vi "lab3.vi"() -> ()   [LabVIEW 2019]
uses:
  <vilib>/imath/engines/lvmath2/RunTimeEngine/BuiltInFunctions/iir_elliptic/NIMS_[2o]_iir_elliptic(I32,DBL2,V,Str).vi
  <vilib>/imath/engines/lvmath2/RunTimeEngine/ErrorHandling/NIMS_Create Error From Enums.vi
  <vilib>/imath/engines/lvmath/Plug In/Control Design/BuiltInFunctions/tf/NIMS_CD_tf(num,den,Ts).vi
  <vilib>/imath/engines/lvmath2/RunTimeEngine/BuiltInFunctions/iir_elliptic/NIMS_[3o]_iir_elliptic(I32,DBL2,V,Str).vi
  <vilib>/imath/engines/lvmath/Plug In/Control Design/BuiltInFunctions/zpk/NIMS_CD_zpk(zeros,poles,k,Ts).vi
  <vilib>/imathl/engines/lvmath/Functions/Error Handling/Create Error.vi
  <vilib>/imath/engines/lvmath2/RunTimeEngine/BuiltInFunctions/iir_elliptic/NIMS_[4o]_iir_elliptic(I32,DBL2,V,Str).vi
  <vilib>/imath/engines/lvmath/Plug In/Control Design/BuiltInFunctions/ss/NIMS_CD_ss(A,B,C,D).vi
  <vilib>/imath/engines/lvmath2/RunTimeEngine/NodeEndStatement/NIMS_NodeEndStatement_Output.vi
  <instcachedir>/0/NIMS_NodeEndStatement_Output_53EC0D466D134D7ABD903AC30B43404B.lvgen/NIMS_NodeEndStatement_Output_53EC0D466D134D7ABD903AC30B43404B_011.vi
  <instcachedir>/0/NIMS_NodeEndStatement_Output_53EC0D466D134D7ABD903AC30B43404B.lvgen/NIMS_NodeEndStatement_Output_53EC0D466D134D7ABD903AC30B43404B_010.vi
  <instcachedir>/0/NIMS_NodeEndStatement_Output_53EC0D466D134D7ABD903AC30B43404B.lvgen/NIMS_NodeEndStatement_Output_53EC0D466D134D7ABD903AC30B43404B_009.vi
  <vilib>/imath/engines/lvmath2/RunTimeEngine/ErrorHandling/NIMS_Finalize Error.vi
  <vilib>/addons/Control Design/_Time Response Analysis/Time Response.llb/Time Response subVI/cd_Step Response (State-Space).vi
  <vilib>/addons/Control Design/_Frequency Response Analysis/Frequency Response.llb/Frequency Response subVI/cd_Bode (State Space).vi
  <vilib>/addons/Control Design/_Utility/Model Viewer.llb/Model Viewer SubVI/cd_Draw State-Space Equation (SS).vi
  <vilib>/addons/Control Design/_Frequency Response Analysis/Frequency Response.llb/Frequency Response subVI/cd_Bode (Zero-Pole-Gain).vi
  <vilib>/addons/Control Design/_Time Response Analysis/Time Response.llb/Time Response subVI/cd_Step Response (Zero-Pole-Gain).vi
  <vilib>/addons/Control Design/_Utility/Model Viewer.llb/Model Viewer SubVI/cd_Draw Zero-Pole-Gain Equation (ZPK).vi
  <vilib>/addons/Control Design/_Frequency Response Analysis/Frequency Response.llb/Frequency Response subVI/cd_Bode (Transfer Function).vi
  <vilib>/addons/Control Design/_Time Response Analysis/Time Response.llb/Time Response subVI/cd_Step Response (Transfer Function).vi
  <vilib>/addons/Control Design/_Utility/Model Viewer.llb/Model Viewer SubVI/cd_Draw Transfer Function Equation (TF).vi
  <vilib>/addons/Control Design/_Utility/NI_CD_Model Viewer.lvlib
  <vilib>/addons/Control Design/_Time Response Analysis/NI_CD_Time Response.lvlib
  <vilib>/addons/Control Design/_Frequency Response Analysis/NI_CD_Frequency Response.lvlib
panel:
  out "Нули, полюса и коэффициент усиления (zpk)":picture
  out "Реакция на ступенчатое воздействие":cluster{"time":dbl[], dbl[]}[](graph)
  out "Реакция АЧХ, реализованных различным способом":cluster{"time":dbl[], dbl[]}[](graph)
  out "АЧХ":cluster{"time":dbl[], dbl[]}[](graph)
  out "Погрешность реакции на ступенчатое воздействие":cluster{"time":dbl[], dbl[]}[](graph)
  out "Передаточная функция":picture
  out "Модель в пространстве состояний":picture
  in  "dbp":dbl
  in  "n":dbl
  in  "dbs":dbl
  in  "w":dbl
  in  "Time Range":cluster{"t0":dbl, "dt":dbl, "tf":dbl}
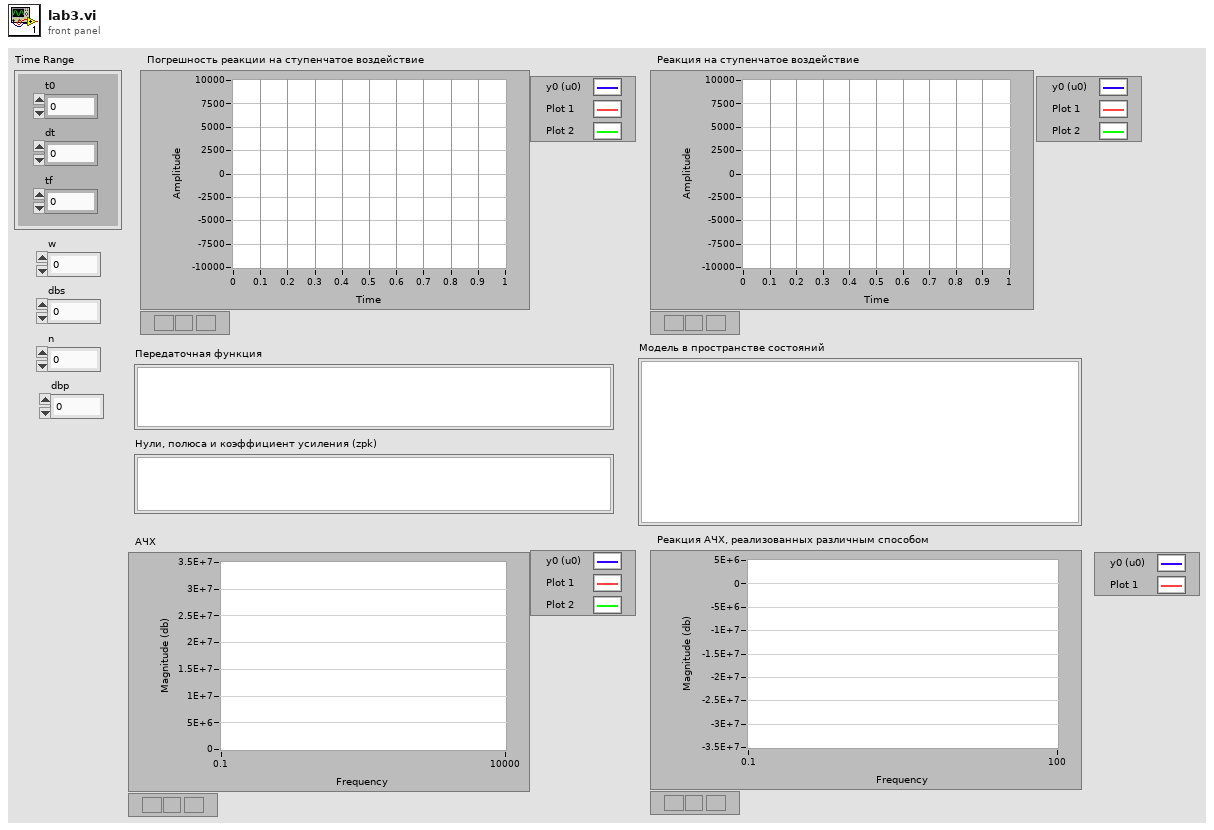
[diagram p1: front panel]
types:
  T1 = typedef "NI_LinSys_Model Typedefs.lvlib/CD Transfer Function Model (MIMO).ctl" = cluster{"properties":T2, "transfer function(s)":T3[][]}
  T2 = typedef "NI_LinSys_Model Typedefs.lvlib/CD General Elements.ctl" = cluster{"Model name":string, "Input names":string[], "Output names":string[], "Input Delays":dbl[], "Output Delays":dbl[], "Sampling Time":dbl, "Notes":string}
  T3 = typedef "NI_LinSys_Model Typedefs.lvlib/CD Transfer Function Model (SISO).ctl" = cluster{"Numerator":dbl[], "Denominator":dbl[], "delay":dbl}
  T4 = typedef "NI_LinSys_Model Typedefs.lvlib/CD Zero-Pole-Gain Model (MIMO).ctl" = cluster{"properties":T2, "zero-pole-gain(s)":T5[][]}
  T5 = typedef "NI_LinSys_Model Typedefs.lvlib/CD Zero-Pole-Gain Model (SISO).ctl" = cluster{"Gain":dbl, "Zeros":cdb[], "Poles":cdb[], "delay":dbl}
  T6 = typedef "NI_LinSys_Model Typedefs.lvlib/CD State Space Model (MIMO).ctl" = cluster{"properties":T2, "A":dbl[][], "B":dbl[][], "C":dbl[][], "D":dbl[][], "StateNames":string[], "Transport Delay":dbl[][]}
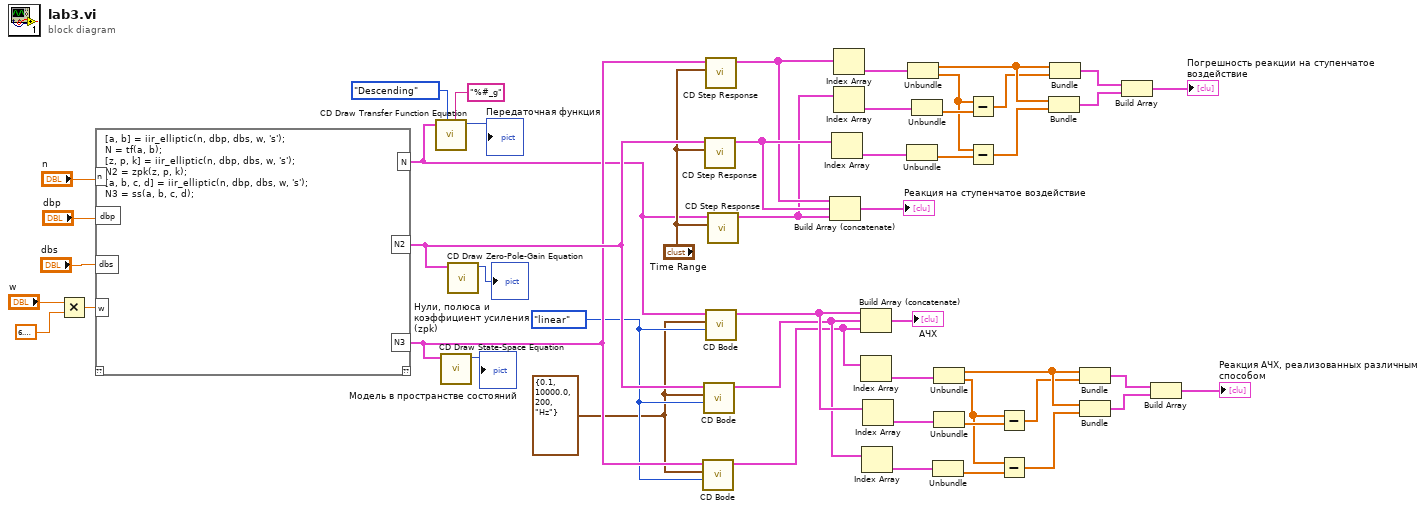
[diagram p0: block diagram]
diagram:
  w35 = enum16{"linear"}."linear"
  w34 = cluster{dbl, dbl, i32, enum16{"Hz"}} {0.1, 10000.0, 200, enum."Hz"} ("Frequency Range")
  n1 = Multiply(x="w", y=6.283185307179586) -> (x*y=w48:dbl)
  n2 = mathscript code="[a, b] = iir_elliptic(n, dbp, dbs, w, 's');\nN = tf(a, b);\n[z, p, k] = iir_elliptic(n, dbp, dbs, w, 's');\nN2 = zpk(z, p, k);\n[a, b, c, d] = iir_elliptic(n, dbp, dbs, w, 's');\nN3 = ss(a, b, c, d);"("n"="n", "dbp"="dbp", "dbs"="dbs", "w"=w48) -> ("N"=w36:T1, "N2"=w43:T4, "N3"=w37:T6)  [unwired: 1 in, 1 out]
  n3 = call-poly <vilib>:"CD Draw Transfer Function Equation.vi"("Format Coefficients"="%#_g", "Display Format"=enum16{"", "Ascending", "Descending"}."Descending", "Transfer Function Model"=w36) -> ("Equation"=→"Передаточная функция":picture)  [unwired: 6 in, 2 out]
  n4 = call-poly <vilib>:"CD Draw State-Space Equation.vi"("State-Space Model"=w37) -> ("Equation"=→"Модель в пространстве состояний":picture)  [unwired: 8 in, 2 out]
  n5 = call-poly <vilib>:"CD Draw Zero-Pole-Gain Equation.vi"("Zero-Pole-Gain Model"=w43) -> ("Equation"=→"Нули, полюса и коэффициент усиления (zpk)":picture)  [unwired: 8 in, 2 out]
  n6 = call-poly <vilib>:"CD Bode.vi"("Magnitude Scale"=w35, "Frequency Range"=w34, "State-Space Model"=w37) -> ("Bode Magnitude"=w22:cluster{"W":dbl[], "Magnitude":dbl[]}[])  [unwired: 4 in, 4 out]
  n7 = call-poly <vilib>:"CD Bode.vi"("Magnitude Scale"=w35, "Frequency Range"=w34, "Zero-Pole-Gain Model"=w43) -> ("Bode Magnitude"=w23:cluster{"W":dbl[], "Magnitude":dbl[]}[])  [unwired: 4 in, 4 out]
  n8 = call-poly <vilib>:"CD Step Response.vi"("Time Range"="Time Range", "Zero-Pole-Gain Model"=w43) -> ("Step Response Graph"=w3:cluster{"time":dbl[], dbl[]}[])  [unwired: 7 in, 2 out]
  n9 = call-poly <vilib>:"CD Step Response.vi"("Time Range"="Time Range", "State-Space Model"=w37) -> ("Step Response Graph"=w2:cluster{"time":dbl[], dbl[]}[])  [unwired: 6 in, 3 out]
  n10 = call-poly <vilib>:"CD Bode.vi"("Magnitude Scale"=w35, "Frequency Range"=w34, "Transfer Function Model"=w36) -> ("Bode Magnitude"=w24:cluster{"W":dbl[], "Magnitude":dbl[]}[])  [unwired: 4 in, 4 out]
  n11 = call-poly <vilib>:"CD Step Response.vi"("Time Range"="Time Range", "Transfer Function Model"=w36) -> ("Step Response Graph"=w1:cluster{"time":dbl[], dbl[]}[])  [unwired: 7 in, 2 out]
  n12 = Build Array (concatenate)(w2, w3, w1) -> (→"Реакция на ступенчатое воздействие":cluster{"time":dbl[], dbl[]}[])
  n13 = Index Array(array=w3) -> (element=w31:cluster{"time":dbl[], dbl[]})  [unwired: 1 in]
  n14 = Index Array(array=w2) -> (element=w33:cluster{"time":dbl[], dbl[]})  [unwired: 1 in]
  n15 = Index Array(array=w1) -> (element=w32:cluster{"time":dbl[], dbl[]})  [unwired: 1 in]
  n16 = Build Array (concatenate)(w24, w23, w22) -> (→"АЧХ":cluster{"W":dbl[], "Magnitude":dbl[]}[])
  n17 = Index Array(array=w22) -> (element=w21:cluster{"W":dbl[], "Magnitude":dbl[]})  [unwired: 1 in]
  n18 = Index Array(array=w23) -> (element=w19:cluster{"W":dbl[], "Magnitude":dbl[]})  [unwired: 1 in]
  n19 = Index Array(array=w24) -> (element=w20:cluster{"W":dbl[], "Magnitude":dbl[]})  [unwired: 1 in]
  n20 = Unbundle(w31) -> (w28:dbl[])  [unwired: 1 out]
  n21 = Unbundle(w33) -> ("time"=w30:dbl[], w27:dbl[])
  n22 = Unbundle(w32) -> (w29:dbl[])  [unwired: 1 out]
  n23 = Unbundle(w19) -> ("Magnitude"=w17:dbl[])  [unwired: 1 out]
  n24 = Unbundle(w21) -> ("W"=w16:dbl[], "Magnitude"=w4:dbl[])
  n25 = Unbundle(w20) -> ("Magnitude"=w18:dbl[])  [unwired: 1 out]
  n26 = Subtract(x=w27, y=w29) -> (x-y=w26:dbl[])
  n27 = Subtract(x=w27, y=w28) -> (x-y=w25:dbl[])
  n28 = Subtract(x=w4, y=w18) -> (x-y=w15:dbl[])
  n29 = Subtract(x=w4, y=w17) -> (x-y=w14:dbl[])
  n30 = Bundle("time"=w30, w25) -> (w12:cluster{"time":dbl[], dbl[]})  [unwired: 1 in]
  n31 = Bundle("time"=w30, w26) -> (w13:cluster{"time":dbl[], dbl[]})  [unwired: 1 in]
  n32 = Bundle("W"=w16, w15) -> (w11:cluster{"W":dbl[], dbl[]})  [unwired: 1 in]
  n33 = Bundle("W"=w16, w14) -> (w10:cluster{"W":dbl[], dbl[]})  [unwired: 1 in]
  n34 = Build Array(w13, w12) -> (→"Погрешность реакции на ступенчатое воздействие":cluster{"time":dbl[], dbl[]}[])
  n35 = Build Array(w11, w10) -> (→"Реакция АЧХ, реализованных различным способом":cluster{"W":dbl[], dbl[]}[])
